vi "Path to Errors File.vi"(8 "Error In":errorcluster) -> (0 "Error Out":errorcluster, 3 "Path to Errors File":path)   [LabVIEW 2019]
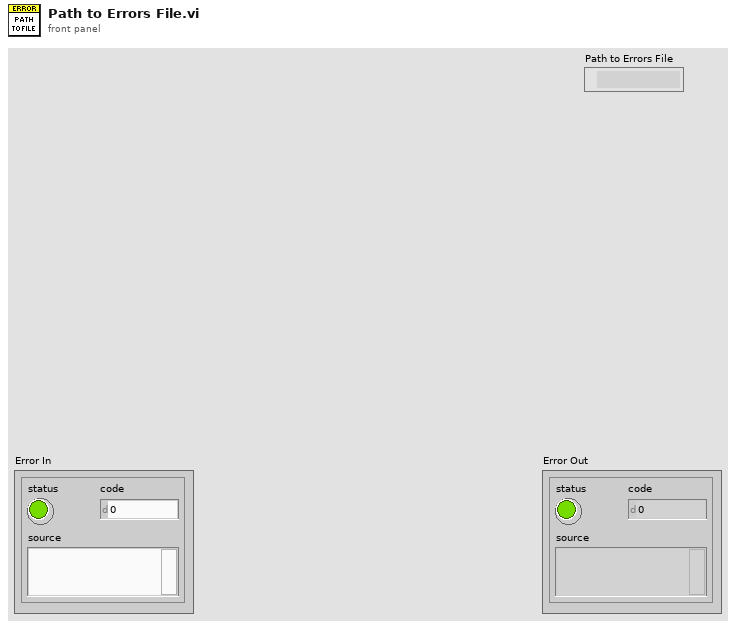
[diagram p1: front panel]
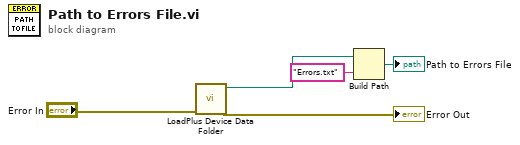
[diagram p0: block diagram]
diagram:
  n1 = call "LoadPlus Device Data Folder.vi"("Error In"="Error In") -> ("Error Out"=→"Error Out":errorcluster, "system directory"=w5:path)  [unwired: 9 in]
  n2 = Build Path(base path=w5, name or relative path="Errors.txt") -> (appended path=→"Path to Errors File":path)
